vi "GV PMT sim.vi"() -> ()   [LabVIEW 2017]
panel:
  out "PMTsim":bool
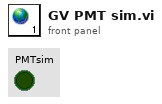
[diagram p1: front panel]
diagram:
